vi "Main.vi"() -> ()   [LabVIEW 2013]
uses:
  <vilib>/Utility/file.llb/Read From Spreadsheet File (DBL).vi
  <vilib>/gmath/NI_Gmath.lvlib
panel:
  out "温度值":dbl[](array[numeric])
  in  "电阻值":dbl[](array[numeric])
  in  "定标文件":string(combo)
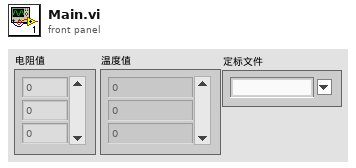
[diagram p1: front panel]
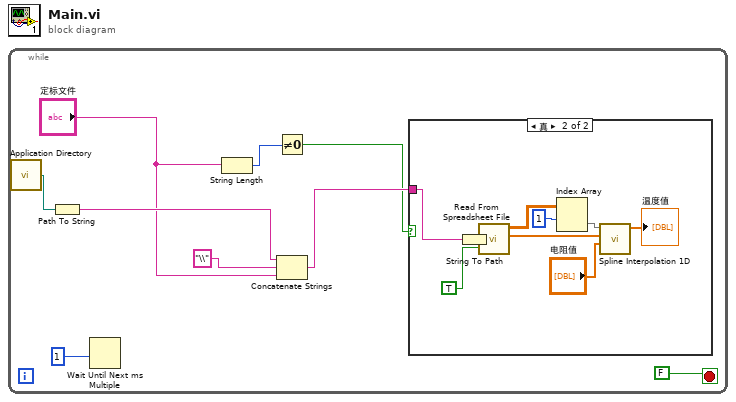
[diagram p0: block diagram]
diagram:
  n1 = while {
    stop <- FALSE stop-if-true
    n2 = call <vilib>:"Application Directory.vi"() -> ("Application Directory"=w9:path)
    n3 = Path To String(path=w9) -> (string=w8:string)
    n4 = Wait Until Next ms Multiple(millisecond multiple=1) -> ()  [unwired: 1 out]
    n5 = String Length(string="定标文件") -> (length=w4:i32)
    n6 = Not Equal To 0?(x=w4) -> (x != 0?=w3:bool)
    n7 = Concatenate Strings(w8, "\\", "定标文件") -> (w6:string)
    n8 = case shown="真" w3 {
      tunnel: w6 -> [_ w10]
      frame False {
      }
      frame True {
        n9 = String To Path(string=w10) -> (path=w16:path)
        n10 = call-poly <vilib>:"Read From Spreadsheet File.vi"("transpose (no:F)"=TRUE, "file path (dialog if empty)"=w16) -> ("first row"=w13:dbl[], "all rows"=w18:dbl[][])  [unwired: 5 in, 3 out]
        n11 = Index Array(array=w18, index (row)=1) -> (element=w17:dbl[])  [unwired: 1 in]
        n12 = call <vilib>:"Spline Interpolation 1D.vi"("xi"="电阻值", "X"=w13, "Y"=w17) -> ("yi"=→"温度值":dbl[])  [unwired: 6 in, 2 out]
      }
    }
  }
